vi "Ctrl.Get Tab Control Pos Info.vi"(3 "error in":errorcluster, 4 "Include Tab Height":bool, 5 "TabCtl Ref":refnum<vi>) -> (0 "error out":errorcluster, 1 "Pos Info":T1, 2 "TabCtl Ref Out":refnum<vi>)   [LabVIEW 2024, in "EQMF.lvlib" / "Controls.lvlib"]
uses:
  Controls.lvlib
  Ctrl.Object Position Info.ctl
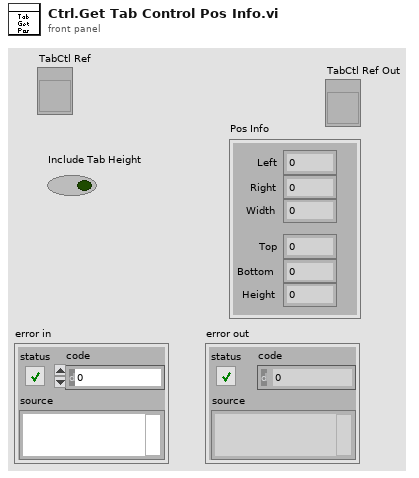
[diagram p1: front panel]
types:
  T1 = typedef "EQMF.lvlib/Controls.lvlib/Ctrl.Object Position Info.ctl" = cluster{"Left":i32, "Right":i32, "Width":i32, "Top":i32, "Bottom":i32, "Height":i32}
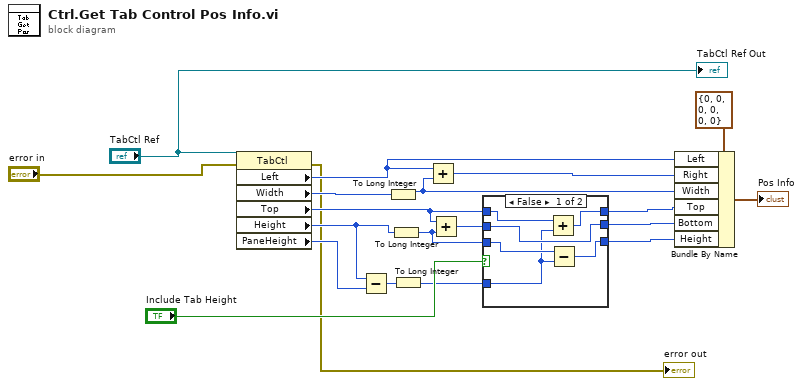
[diagram p0: block diagram]
diagram:
  n1 = property on="Property Node" class="TabCtl"(reference="TabCtl Ref", error in="error in") -> (error out=→"error out":errorcluster, "Left"=w18:i32, "Width"=w11:u32, "Top"=w10:i32, "Height"=w7:u32, "PaneHeight"=w6:u32)  [unwired: 1 out]
  n2 = Subtract(x=w7, y=w6) -> (x-y=w5:u32)
  n3 = To Long Integer(number=w11) -> (32bit integer=w16:i32)
  n4 = To Long Integer(number=w7) -> (32bit integer=w8:i32)
  n5 = To Long Integer(number=w5) -> (32bit integer=w4:i32)
  n6 = Add(x=w18, y=w16) -> (x+y=w17:i32)
  n7 = Add(x=w10, y=w8) -> (x+y=w9:i32)
  n8 = case shown="False" "Include Tab Height" {
    tunnel: w10 -> [w26 w29]
    tunnel: w9 -> [w24 w28]
    tunnel: w8 -> [w22 w27]
    tunnel: [w25 w29] -> w15
    tunnel: [w24 w28] -> w14
    tunnel: [w23 w27] -> w13
    tunnel: w4 -> [w21 _]
    frame False {
      n9 = Add(x=w26, y=w21) -> (x+y=w25:i32)
      n10 = Subtract(x=w22, y=w21) -> (x-y=w23:i32)
    }
    frame True {
    }
  }
  n11 = Bundle By Name(cluster=T1 {"Left"=0, "Right"=0, "Width"=0, "Top"=0, "Bottom"=0, "Height"=0} ("Pos Info"), "Left"=w18, "Right"=w17, "Width"=w16, "Top"=w15, "Bottom"=w14, "Height"=w13) -> (→"Pos Info":T1)
  "TabCtl Ref Out" <- "TabCtl Ref"
